vi "ReadDefaultConfigurationFile.vi"(8 "error in (no error)":errorcluster, 11 "SMO.UI.MAUI in":refnum<class "MAUI.lvclass">) -> (0 "error out":errorcluster, 2 "Default Data":T1, 3 "SMO.UI.MAUI out":refnum<class "MAUI.lvclass">)   [LabVIEW 2019, in "MAUI.lvclass"]
doc: "Reads the framework's default configuration data. The configuration file is located at %PublicApplicationData%\\maui\\maui_framework\\resource\\default.ini."
uses:
  MAUI.lvclass
  Typedefs/DefaultConfiguration.ctl
  <vilib>/Utility/config.llb/NI_LVConfig.lvlib
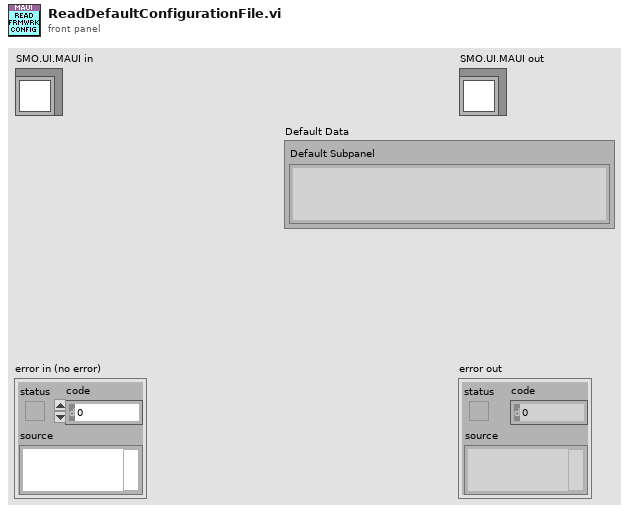
[diagram p1: front panel]
types:
  T1 = typedef "MAUI.lvclass/DefaultConfiguration.ctl" = cluster{"Default Subpanel":string}
  T2 = typedef "NI_LVConfig.lvlib/Config Data RefNum.ctl" = refnum<k1>
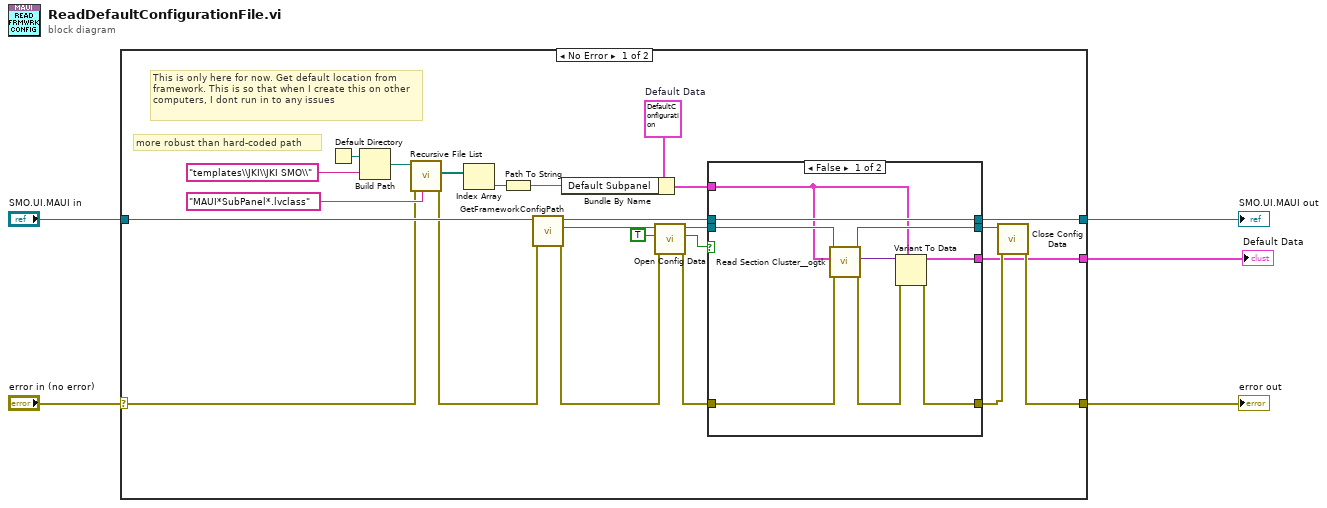
[diagram p0: block diagram]
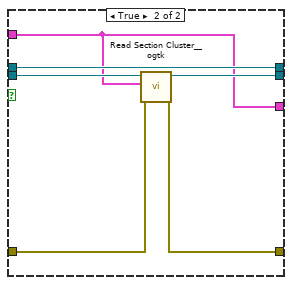
[diagram p2: hidden frame]
diagram:
  n1 = case shown="No Error" "error in (no error)" {
    selector: "error in (no error)" -> [w8 w46]
    tunnel: [w26 w46] -> w4
    tunnel: [w21 w45] -> w2
    tunnel: "SMO.UI.MAUI in" -> [w25 w45]
    tunnel: [w17 _] -> w1
    frame No Error {
      w16 = T1 {"Default Subpanel"="C:\\Program Files (x86)\\National Instruments\\LabVIEW 2020\\templates\\JKI\\JKI SMO\\LevyLab\\SMO.UI.Embedded.Basic.lvclass"}  # Default Data
      # "more robust than hard-coded path"
      # "This is only here for now. Get default location from framework. This is so that when I create this on other computers, I dont run in to any issues"
      n2 = Default Directory() -> (w14:path)
      n3 = Build Path(base path=w14, name or relative path="templates\\JKI\\JKI SMO\\") -> (appended path=w12:path)
      n4 = call <vilib>:"Recursive File List.vi"("pattern"="MAUI*SubPanel*.lvclass", "error in (no error)"=w8, "Folder Path"=w12) -> ("error out"=w7:errorcluster, "All Files in Dir"=w10:path[])  [unwired: 4 in, 3 out]
      n5 = Index Array(array=w10) -> (element=w9:path)  [unwired: 1 in]
      n6 = Path To String(path=w9) -> (string=w6:string)
      n7 = call "GetFrameworkConfigPath.vi"("error in (no error)"=w7, "SMO.UI.MAUI in"=w25) -> ("error out"=w29:errorcluster, "Path"=w23:path, "SMO.UI.MAUI out"=w22:refnum<class "MAUI.lvclass">)  [unwired: 7 in]
      n8 = Bundle By Name(cluster=w16, "Default Subpanel"=w6) -> (w15:T1)
      n9 = call <vilib>:"Open Config Data.vi"("error in (no error)"=w29, "create file if necessary (T)"=TRUE, "configuration file path"=w23) -> ("error out"=w28:errorcluster, "file created?"=w20:bool, "refnum"=w19:T2)  [unwired: 6 in]
      n10 = case shown="False" w20 {
        tunnel: w22 -> [w35 w42]
        tunnel: [w35 w42] -> w21
        tunnel: [w36 w44] -> w27
        tunnel: w28 -> [w38 w43]
        tunnel: w19 -> [w34 w41]
        tunnel: [w33 w40] -> w18
        tunnel: w15 -> [w31 w39]
        tunnel: [w30 w39] -> w17
        frame False {
          n11 = call <userlib>:"Read Section Cluster__ogtk.vi"("error in (no error)"=w38, "Section Formatted Cluster Type"=w31, "refnum"=w34) -> ("error out"=w37:errorcluster, "Section Formatted Cluster"=w32:variant, "dup refnum"=w33:T2)  [unwired: 4 in, 2 out]
          n12 = Variant To Data(error in=w37, type=w31, Variant=w32) -> (data=w30:T1, error out=w36:errorcluster)
        }
        frame True {
          n13 = call <userlib>:"Read Section Cluster__ogtk.vi"("error in (no error)"=w43, "Section Formatted Cluster Type"=w39, "refnum"=w41) -> ("error out"=w44:errorcluster, "dup refnum"=w40:T2)  [unwired: 4 in, 3 out]
        }
      }
      n14 = call <vilib>:"Close Config Data.vi"("error in (no error)"=w27, "refnum"=w18) -> ("error out"=w26:errorcluster)  [unwired: 8 in, 1 out]
    }
    frame Error {
    }
  }
  "error out" <- w4
  "SMO.UI.MAUI out" <- w2
  "Default Data" <- w1
